vi "外观 1.vi"(0 "Data In":T6=enum."集成式多参数" caption="数据输入", 2 "Display State In":T3={"模块启用"={"原位多参数"=FALSE, "集成式多参数"=FALSE, "营养盐"=FALSE}, "模块名称"={"原位多参数"="环境动力", "集成式多参数"="氨氮", "营养盐"="总磷"}} caption="显示状态输入", 3 "Container State":T5 caption="容器状态") -> (6 "Data Out":T6=enum."集成式多参数" caption="数据输出", 7 "Display State Out":T3={"模块启用"={"原位多参数"=FALSE, "集成式多参数"=FALSE, "营养盐"=FALSE}, "模块名称"={"原位多参数"="环境动力", "集成式多参数"="氨氮", "营养盐"="总磷"}} caption="显示状态输出", 8 "Action":T2 caption="动作")   [LabVIEW 2016, in "运维调试菜单.xctl"]
uses:
  <vilib>/_xctls/Container State.ctl
  <vilib>/_xctls/Action.ctl
  <vilib>/Utility/miscctls.llb/LVPointTypeDef.ctl
  <vilib>/_xctls/XControlSupport.lvlib
panel:
  in  "单选按钮":T1
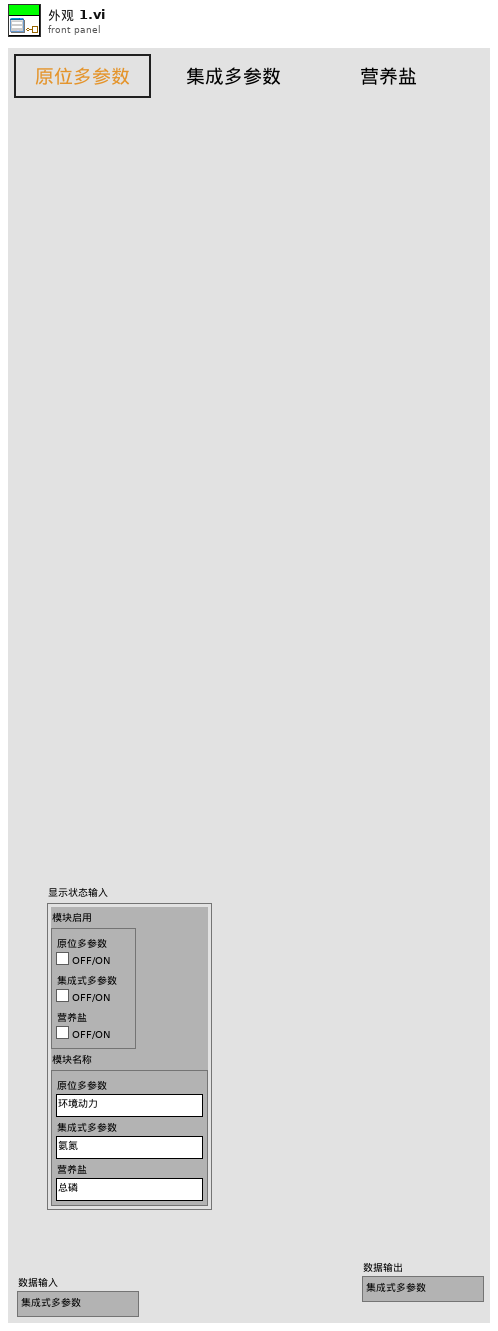
[diagram p1: front panel]
types:
  T1 = typedef "运维调试菜单.xctl/控件外观.ctl" = enum32{"原位多参数", "集成式多参数", "营养盐"}
  T2 = typedef "XControlSupport.lvlib/Action.ctl" = cluster{"Data Changed?":bool, "State Changed?":bool, "Action Name":string}
  T3 = typedef "运维调试菜单.xctl/状态 1.ctl" = cluster{"模块启用":T4, "模块名称":cluster{"原位多参数":string, "集成式多参数":string, "营养盐":string}}
  T4 = typedef "运维调试菜单.xctl/模块启用.ctl" = cluster{"原位多参数":bool, "集成式多参数":bool, "营养盐":bool}
  T5 = typedef "XControlSupport.lvlib/Container State.ctl" = cluster{"Indicator?":bool, "Run Mode?":bool, " Refnum":refnum<vi>}
  T6 = typedef "运维调试菜单.xctl/数据 1.ctl" = enum16{"原位多参数", "集成式多参数", "营养盐"}
  T7 = typedef "LVPointTypeDef.ctl" = cluster{"Horizontal":i16, "Vertical":i16}
  T8 = cluster{"原位多参数":string, "集成式多参数":string, "营养盐":string}
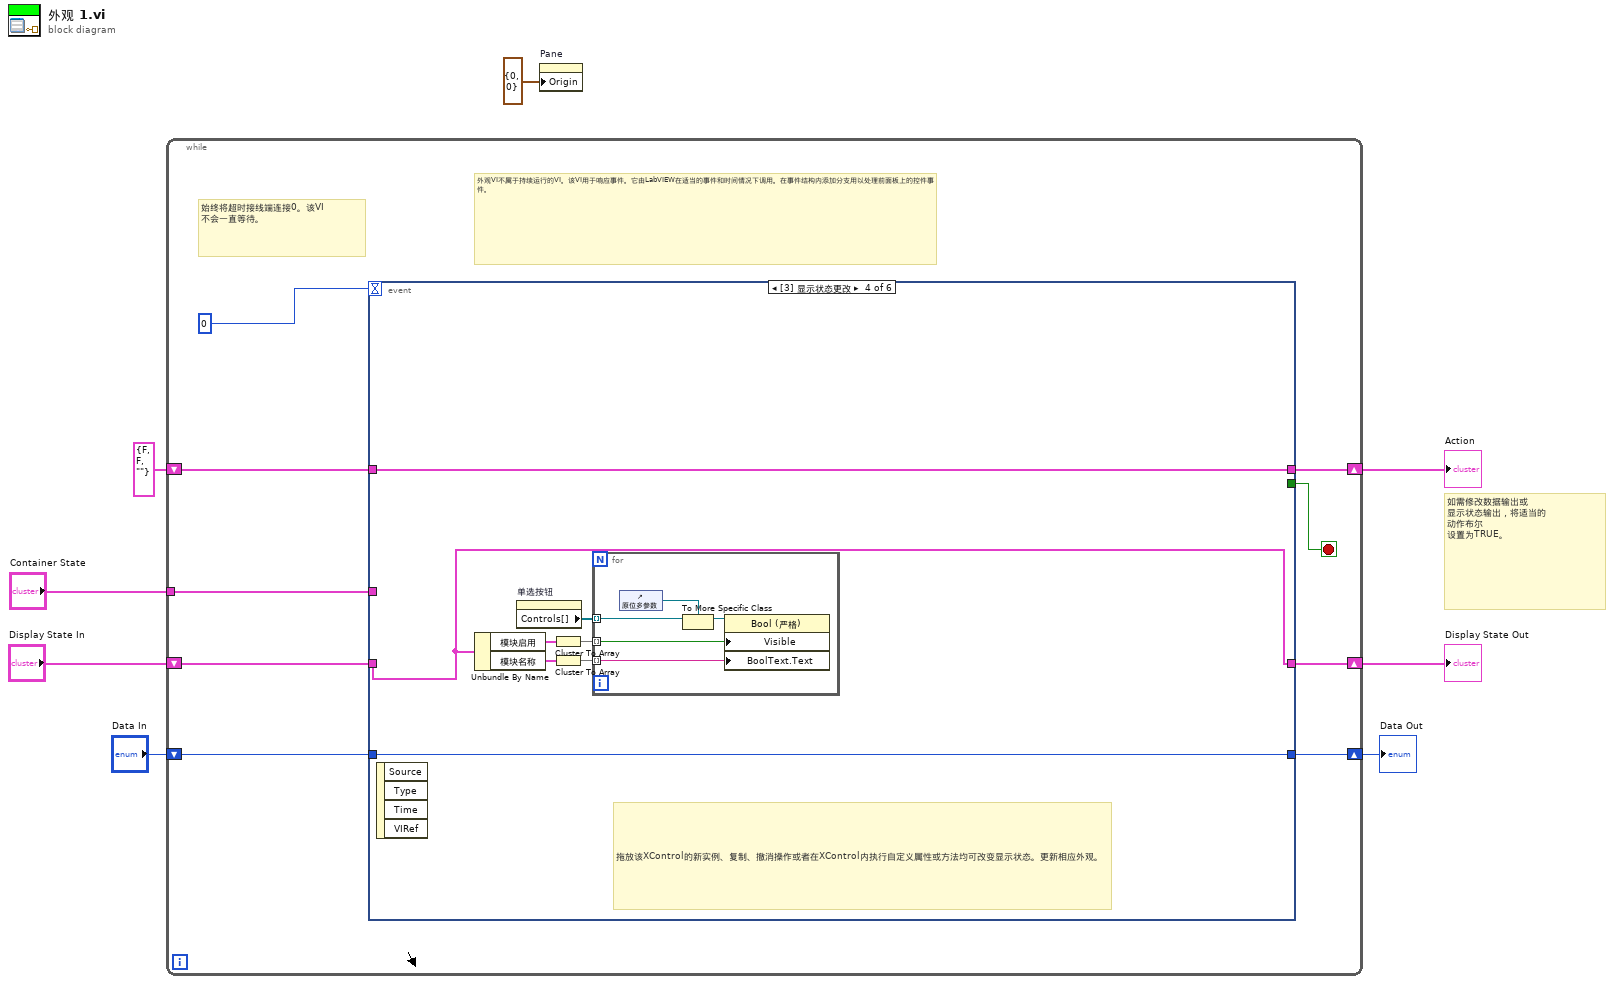
[diagram p0: block diagram]
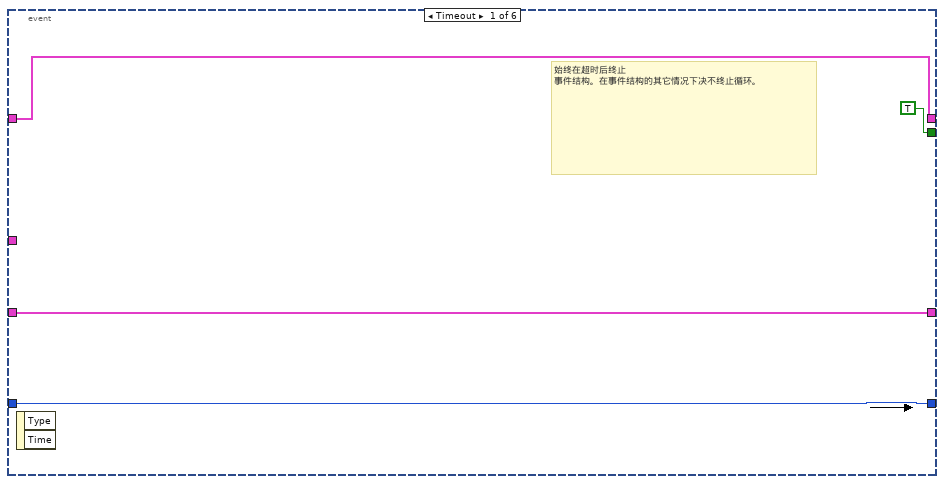
[diagram p2: hidden frame]
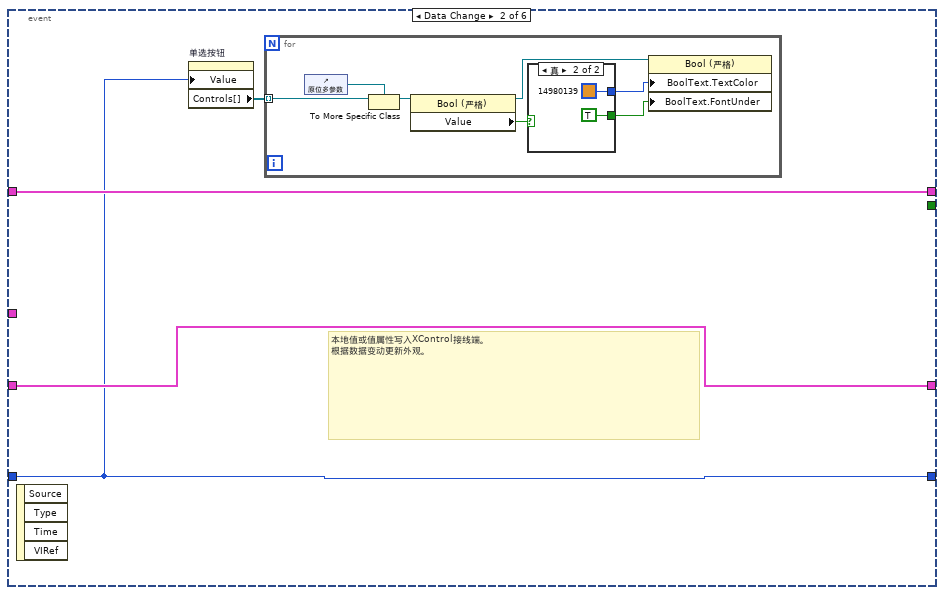
[diagram p3: hidden frame]
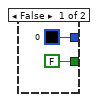
[diagram p4: hidden frame]
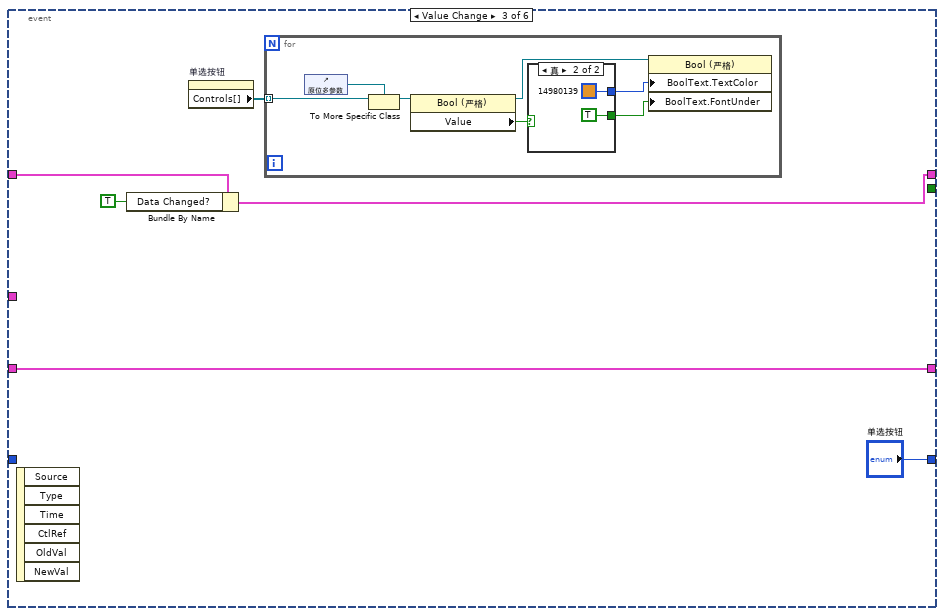
[diagram p5: hidden frame]
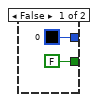
[diagram p6: hidden frame]
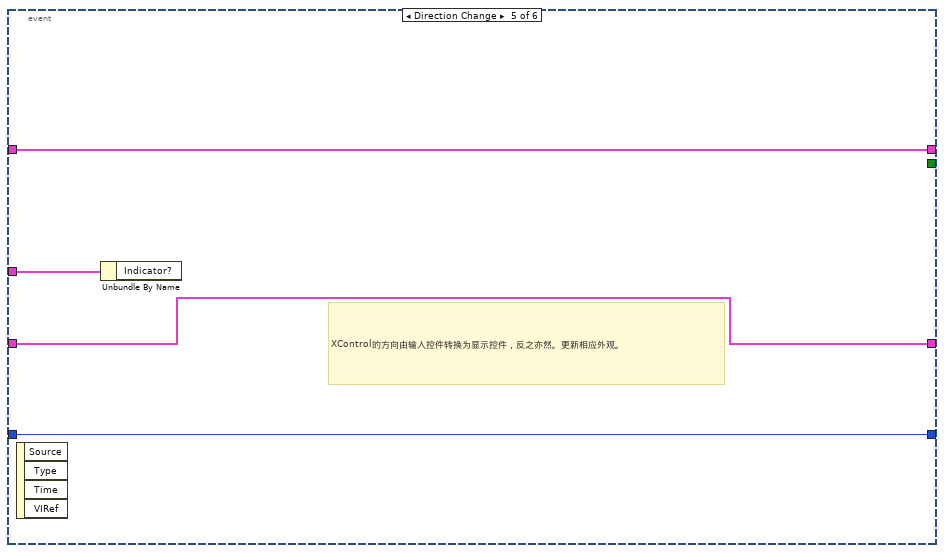
[diagram p7: hidden frame]
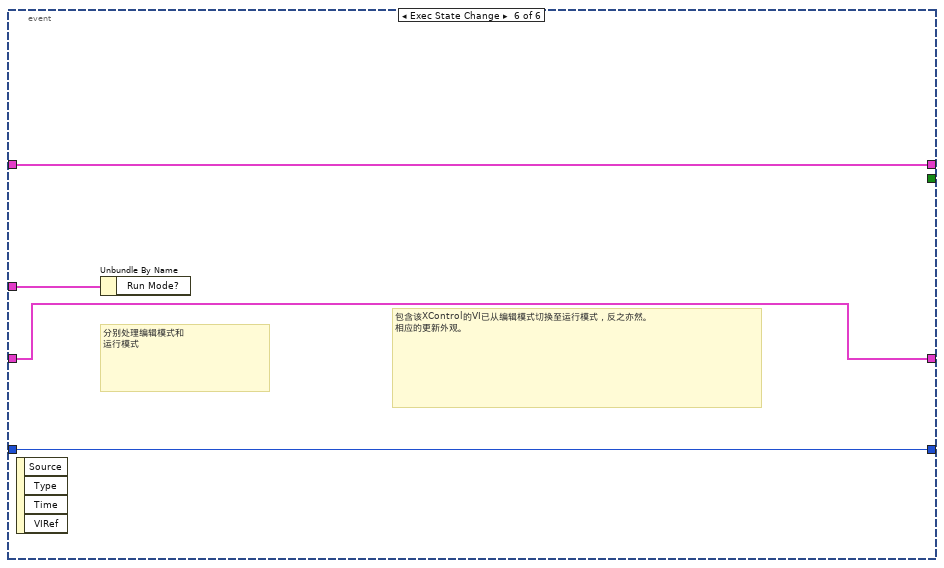
[diagram p8: hidden frame]
diagram:
  # "如需修改数据输出或\n显示状态输出，将适当的\n动作布尔\n设置为TRUE。"
  n1 = while {
    shift-right: [w16] -> w5
    shift-left: "Display State In" -> [w17]
    tunnel: "Container State" -> [w13]
    shift-right: [w11] -> w8
    shift-left: "Data In" -> [w12]
    shift-right: [w9] -> w3
    shift-left: T2 {"Data Changed?"=FALSE, "State Changed?"=FALSE, "Action Name"=""} ("Action") -> [w10]
    stop <- w15 stop-if-true
    # "外观VI不属于持续运行的VI。该VI用于响应事件。它由LabVIEW在适当的事件和时间情况下调用。在事件结构内添加分支用以处理前面板上的控件事件。"
    # "始终将超时接线端连接0。该VI\n不会一直等待。"
    n2 = event shown="[3] 显示状态更改" {
      selector: _ -> [_ _ _ _ _ _]
      dyn-events: _ -> [_ _ _ _ _ _]
      timeout: 0 -> [_ _ _ _ _ _]
      tunnel: w17 -> [w19 w25 w42 w60 w69 w71]
      tunnel: [w19 w25 w42 w60 w69 w71] -> w16
      tunnel: [TRUE _ _ _ _ _] -> w15
      tunnel: w13 -> [_ _ _ _ w70 w74]
      tunnel: w12 -> [w18 w22 _ w54 w68 w73]
      tunnel: [w18 w22 "单选按钮" w54 w68 w73] -> w11
      tunnel: [w20 w24 w40 w61 w67 w72] -> w9
      tunnel: w10 -> [w20 w24 w41 w61 w67 w72]
      event Timeout {
        # "始终在超时后终止\n事件结构。在事件结构的其它情况下决不终止循环。"
        n3 = event-data() -> ()  [unwired: 1 in, 2 out]
      }
      event Data Change {
        # "本地值或值属性写入XControl接线端。\n根据数据变动更新外观。"
        n4 = event-data() -> ()  [unwired: 1 in, 4 out]
        n5 = property on="单选按钮" class="RadioBtnsControl (严格)"("Value"=w22) -> ("Controls[]"=w23:refnum<vi>[])  [unwired: 2 in, 2 out]
        n6 = for {
          tunnel: w23 -> [w32] mode=indexing
          n7 = control-ref of="原位多参数"() -> (w26:refnum<vi>)
          n8 = To More Specific Class(target class=w26, reference=w32) -> (specific class reference=w31:refnum<vi>)  [unwired: 1 in, 1 out]
          n9 = property class="Bool (严格)"(reference=w31) -> (reference out=w30:refnum<vi>, "Value"=w29:bool)  [unwired: 1 in, 1 out]
          n10 = case shown="真" w29 {
            tunnel: [u32 0 u32 14980139] -> w28
            tunnel: [FALSE ("布尔文本.字体:下划线") TRUE ("布尔文本.字体:下划线")] -> w27
            frame False {
            }
            frame True {
            }
          }
          n11 = property class="Bool (严格)"(reference=w30, "BoolText.TextColor"=w28, "BoolText.FontUnder"=w27) -> ()  [unwired: 1 in, 2 out]
        }
      }
      event Value Change {
        n12 = event-data() -> ()  [unwired: 1 in, 6 out]
        n13 = Bundle By Name(cluster=w41, "Data Changed?"=TRUE) -> (w40:T2)
        n14 = property on="单选按钮" class="RadioBtnsControl (严格)"() -> ("Controls[]"=w37:refnum<vi>[])  [unwired: 2 in, 2 out]
        n15 = for {
          tunnel: w37 -> [w49] mode=indexing
          n16 = control-ref of="原位多参数"() -> (w43:refnum<vi>)
          n17 = To More Specific Class(target class=w43, reference=w49) -> (specific class reference=w48:refnum<vi>)  [unwired: 1 in, 1 out]
          n18 = property class="Bool (严格)"(reference=w48) -> (reference out=w47:refnum<vi>, "Value"=w46:bool)  [unwired: 1 in, 1 out]
          n19 = case shown="真" w46 {
            tunnel: [u32 0 u32 14980139] -> w45
            tunnel: [FALSE ("布尔文本.字体:下划线") TRUE ("布尔文本.字体:下划线")] -> w44
            frame False {
            }
            frame True {
            }
          }
          n20 = property class="Bool (严格)"(reference=w47, "BoolText.TextColor"=w45, "BoolText.FontUnder"=w44) -> ()  [unwired: 1 in, 2 out]
        }
      }
      event Display State Change {
        # "拖放该XControl的新实例、复制、撤消操作或者在XControl内执行自定义属性或方法均可改变显示状态。更新相应外观。"
        n21 = event-data() -> ()  [unwired: 1 in, 4 out]
        n22 = Unbundle By Name(w60) -> ("模块启用"=w58:T4, "模块名称"=w56:T8)
        n23 = property on="单选按钮" class="RadioBtnsControl (严格)"() -> ("Controls[]"=w59:refnum<vi>[])  [unwired: 2 in, 2 out]
        n24 = Cluster To Array(cluster=w58) -> (array=w57:bool[])
        n25 = Cluster To Array(cluster=w56) -> (array=w55:string[])
        n26 = for {
          tunnel: w59 -> [w66] mode=indexing
          tunnel: w57 -> [w63] mode=indexing
          tunnel: w55 -> [w62] mode=indexing
          n27 = control-ref of="原位多参数"() -> (w64:refnum<vi>)
          n28 = To More Specific Class(target class=w64, reference=w66) -> (specific class reference=w65:refnum<vi>)  [unwired: 1 in, 1 out]
          n29 = property class="Bool (严格)"(reference=w65, "Visible"=w63, "BoolText.Text"=w62) -> ()  [unwired: 1 in, 2 out]
        }
      }
      event Direction Change {
        # "XControl的方向由输入控件转换为显示控件，反之亦然。更新相应外观。"
        n30 = event-data() -> ()  [unwired: 1 in, 4 out]
        n31 = Unbundle By Name(w70) -> ()  [unwired: 1 out]
      }
      event Exec State Change {
        # "包含该XControl的VI已从编辑模式切换至运行模式，反之亦然。\n相应的更新外观。"
        # "分别处理编辑模式和\n运行模式"
        n32 = event-data() -> ()  [unwired: 1 in, 4 out]
        n33 = Unbundle By Name(w74) -> ()  [unwired: 1 out]
      }
    }
  }
  "Display State Out" <- w5
  "Data Out" <- w8
  "Action" <- w3
  n34 = property on="Pane" class="Pane"("Origin"=T7 {"Horizontal"=0, "Vertical"=0} ("原点")) -> ()  [unwired: 2 in, 2 out]
